vi "set operation mode.vi"(8 "error in (no error)":errorcluster, 11 "CCDCamera in":refnum<class "iKon-L.lvclass">) -> (0 "error out":errorcluster, 3 "CCDCamera out":refnum<class "iKon-L.lvclass">)   [LabVIEW 2018, in "iKon-L.lvclass"]
doc: "Set the camera configuration\n\nThis function records the given operating parameters in the camera. However, the parameters will only bewritten if their last value is different from the most recent one."
uses:
  iKon-L.lvclass
panel:
  out "x != y? 2":T1
  out "x != y?":T2
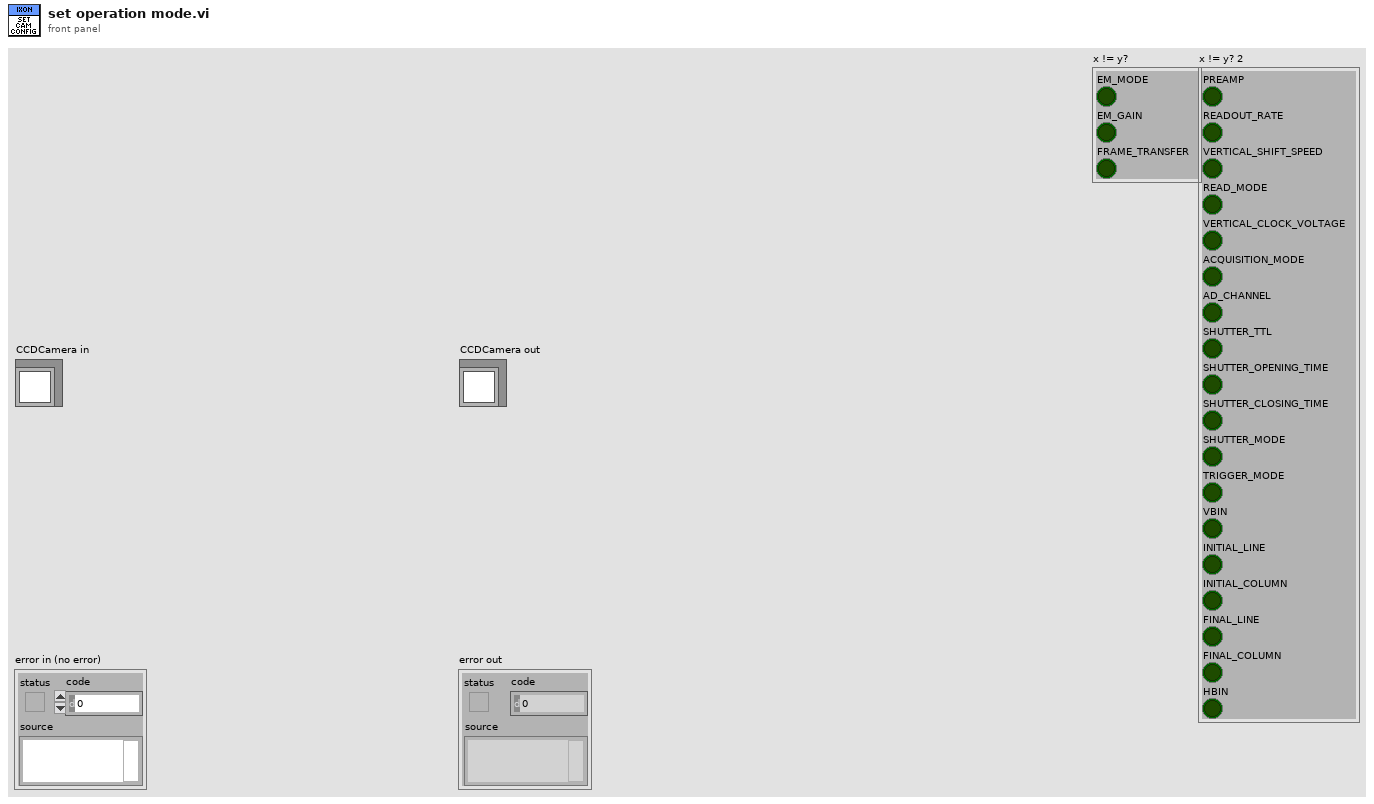
[diagram p1: front panel]
types:
  T1 = cluster{"PREAMP":bool, "READOUT_RATE":bool, "VERTICAL_SHIFT_SPEED":bool, "READ_MODE":bool, "VERTICAL_CLOCK_VOLTAGE":bool, "ACQUISITION_MODE":bool, "AD_CHANNEL":bool, "SHUTTER_TTL":bool, "SHUTTER_OPENING_TIME":bool, "SHUTTER_CLOSING_TIME":bool, "SHUTTER_MODE":bool, "TRIGGER_MODE":bool, "VBIN":bool, "INITIAL_LINE":bool, "INITIAL_COLUMN":bool, "FINAL_LINE":bool, "FINAL_COLUMN":bool, "HBIN":bool}
  T2 = cluster{"EM_MODE":bool, "EM_GAIN":bool, "FRAME_TRANSFER":bool}
  T3 = cluster{"PREAMP":u16, "READOUT_RATE":u16, "VERTICAL_SHIFT_SPEED":u16, "READ_MODE":u16, "VERTICAL_CLOCK_VOLTAGE":u16, "ACQUISITION_MODE":u16, "AD_CHANNEL":u16, "SHUTTER_TTL":u16, "SHUTTER_OPENING_TIME":u16, "SHUTTER_CLOSING_TIME":u16, "SHUTTER_MODE":u16, "TRIGGER_MODE":u16, "VBIN":u16, "INITIAL_LINE":u16, "INITIAL_COLUMN":u16, "FINAL_LINE":u16, "FINAL_COLUMN":u16, "HBIN":u16}
  T4 = cluster{"EM_MODE":u16, "EM_GAIN":u16, "FRAME_TRANSFER":bool}
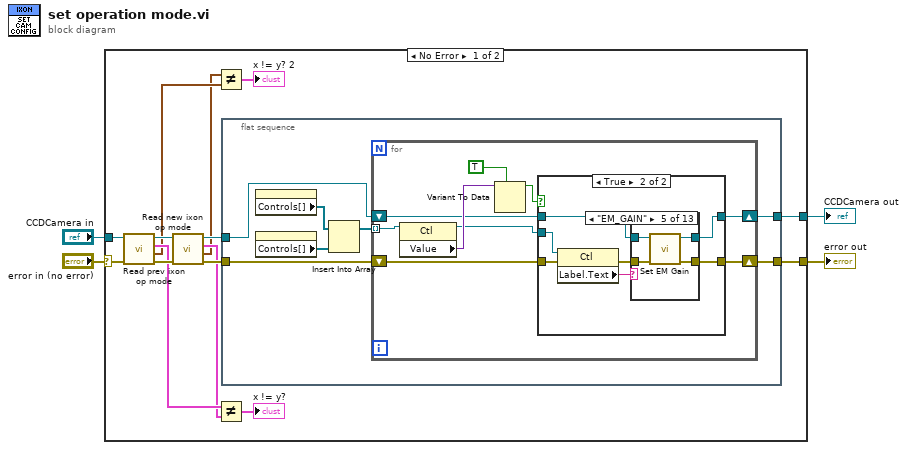
[diagram p0: block diagram]
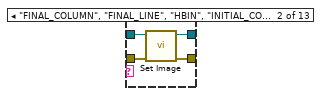
[diagram p4: hidden frame]
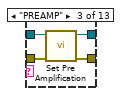
[diagram p5: hidden frame]
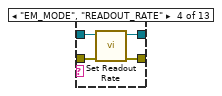
[diagram p6: hidden frame]
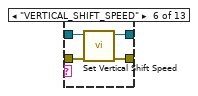
[diagram p7: hidden frame]
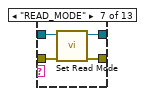
[diagram p8: hidden frame]
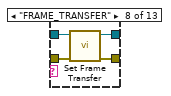
[diagram p9: hidden frame]
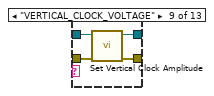
[diagram p10: hidden frame]
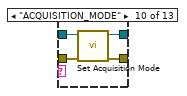
[diagram p11: hidden frame]
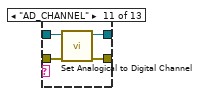
[diagram p12: hidden frame]
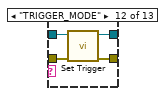
[diagram p13: hidden frame]
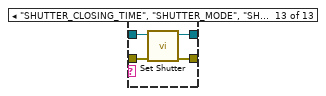
[diagram p14: hidden frame]
diagram:
  n1 = case shown="No Error" "error in (no error)" {
    selector: "error in (no error)" -> [w16 w95]
    tunnel: [w18 w95] -> w4
    tunnel: [w17 w94] -> w3
    tunnel: "CCDCamera in" -> [w15 w94]
    frame No Error {
      n2 = call-dynamic "Read prev ixon op mode.vi"("error in (no error)"=w16, "Sim_Ixon_Ultra in"=w15) -> ("error out"=w13:errorcluster, "prev operation mode"=w7:T3, "prev ixon op mode"=w10:T4, "Sim_Ixon_Ultra out"=w14:refnum<class "iKon-L.lvclass">)  [unwired: 6 in]
      n3 = call-dynamic "Read new ixon op mode.vi"("error in (no error)"=w13, "Sim_Ixon_Ultra in"=w14) -> ("error out"=w12:errorcluster, "new operation mode"=w6:T3, "new ixon op mode"=w9:T4, "Sim_Ixon_Ultra out"=w11:refnum<class "iKon-L.lvclass">)  [unwired: 6 in]
      n4 = Not Equal?(x=w6, y=w7) -> (x != y?=→"x != y? 2":T1)
      n5 = Not Equal?(x=w10, y=w9) -> (x != y?=→"x != y?":T2)
      n6 = flat-sequence {
        tunnel: w12 -> [w22]
        tunnel: [w25] -> w18
        tunnel: w11 -> [w24]
        tunnel: [w23] -> w17
        frame #0 {
          n7 = property on="x != y?" class="Clust (strict)"() -> ("Controls[]"=w20:refnum<vi>[])  [unwired: 2 in, 2 out]
          n8 = property on="x != y? 2" class="Clust (strict)"() -> ("Controls[]"=w19:refnum<vi>[])  [unwired: 2 in, 2 out]
          n9 = Insert Into Array(array=w20, new element=w19) -> (w21:refnum<vi>[])  [unwired: 1 in]
          n10 = for {
            shift-right: [w28] -> w25
            shift-left: w22 -> [w34]
            shift-right: [w29] -> w23
            shift-left: w24 -> [w30]
            tunnel: w21 -> [w27] mode=indexing
            n11 = property class="Ctl"(reference=w27) -> (reference out=w26:refnum<vi>, "Value"=w33:variant)  [unwired: 1 in, 1 out]
            n12 = Variant To Data(type=TRUE, Variant=w33) -> (data=w31:bool)  [unwired: 1 in, 1 out]
            n13 = case shown="True" w31 {
              tunnel: [w36 w38] -> w28
              tunnel: w34 -> [w36 w42]
              tunnel: w30 -> [w35 w41]
              tunnel: [w35 w40] -> w29
              tunnel: w26 -> [_ w37]
              frame False {
              }
              frame True {
                n14 = property class="Ctl"(reference=w37, error in=w42) -> (error out=w39:errorcluster, "Label.Text"=w43:string)  [unwired: 1 out]
                n15 = case shown="\"EM_GAIN\"" w43 {
                  tunnel: w41 -> [w45 w49 w53 w56 w61 w65 w69 w73 w76 w81 w85 w88 w93]
                  tunnel: [w45 w48 w52 w57 w60 w64 w68 w72 w77 w80 w84 w89 w92] -> w40
                  tunnel: w39 -> [w44 w47 w51 w55 w59 w63 w67 w71 w75 w79 w83 w87 w91]
                  tunnel: [w44 w46 w50 w54 w58 w62 w66 w70 w74 w78 w82 w86 w90] -> w38
                  frame "False", Default {
                  }
                  frame "FINAL_COLUMN", "FINAL_LINE", "HBIN", "INITIAL_COLUMN", "INITIAL_LINE", "VBIN" {
                    n16 = call-dynamic "Set Image.vi"("error in (no error)"=w47, "CCDCamera in"=w49) -> ("error out"=w46:errorcluster, "CCDCamera out"=w48:refnum<class "iKon-L.lvclass">)  [unwired: 8 in]
                  }
                  frame "PREAMP" {
                    n17 = call-dynamic "Set Pre Amplification.vi"("error in (no error)"=w51, "CCDCamera in"=w53) -> ("error out"=w50:errorcluster, "CCDCamera out"=w52:refnum<class "iKon-L.lvclass">)  [unwired: 8 in]
                  }
                  frame "EM_MODE", "READOUT_RATE" {
                    n18 = call-dynamic "Set Readout Rate.vi"("error in (no error)"=w55, "CCDCamera in"=w56) -> ("error out"=w54:errorcluster, "CCDCamera out"=w57:refnum<class "iKon-L.lvclass">)  [unwired: 8 in]
                  }
                  frame "EM_GAIN" {
                    n19 = call-dynamic "Set EM Gain.vi"("error in (no error)"=w59, "CCDCamera in"=w61) -> ("error out"=w58:errorcluster, "CCDCamera out"=w60:refnum<class "iKon-L.lvclass">)  [unwired: 8 in]
                  }
                  frame "VERTICAL_SHIFT_SPEED" {
                    n20 = call-dynamic "Set Vertical Shift Speed.vi"("error in (no error)"=w63, "CCDCamera in"=w65) -> ("error out"=w62:errorcluster, "CCDCamera out"=w64:refnum<class "iKon-L.lvclass">)  [unwired: 8 in]
                  }
                  frame "READ_MODE" {
                    n21 = call-dynamic "Set Read Mode.vi"("error in (no error)"=w67, "CCDCamera in"=w69) -> ("error out"=w66:errorcluster, "CCDCamera out"=w68:refnum<class "iKon-L.lvclass">)  [unwired: 8 in]
                  }
                  frame "FRAME_TRANSFER" {
                    n22 = call-dynamic "Set Frame Transfer.vi"("error in (no error)"=w71, "CCDCamera in"=w73) -> ("error out"=w70:errorcluster, "CCDCamera out"=w72:refnum<class "iKon-L.lvclass">)  [unwired: 8 in]
                  }
                  frame "VERTICAL_CLOCK_VOLTAGE" {
                    n23 = call-dynamic "Set Vertical Clock Amplitude.vi"("error in (no error)"=w75, "CCDCamera in"=w76) -> ("error out"=w74:errorcluster, "CCDCamera out"=w77:refnum<class "iKon-L.lvclass">)  [unwired: 8 in]
                  }
                  frame "ACQUISITION_MODE" {
                    n24 = call-dynamic "Set Acquisition Mode.vi"("error in (no error)"=w79, "CCDCamera in"=w81) -> ("error out"=w78:errorcluster, "CCDCamera out"=w80:refnum<class "iKon-L.lvclass">)  [unwired: 8 in]
                  }
                  frame "AD_CHANNEL" {
                    n25 = call-dynamic "Set Analogical to Digital Channel.vi"("error in (no error)"=w83, "CCDCamera in"=w85) -> ("error out"=w82:errorcluster, "CCDCamera out"=w84:refnum<class "iKon-L.lvclass">)  [unwired: 8 in]
                  }
                  frame "TRIGGER_MODE" {
                    n26 = call-dynamic "Set Trigger.vi"("error in (no error)"=w87, "CCDCamera in"=w88) -> ("error out"=w86:errorcluster, "CCDCamera out"=w89:refnum<class "iKon-L.lvclass">)  [unwired: 8 in]
                  }
                  frame "SHUTTER_CLOSING_TIME", "SHUTTER_MODE", "SHUTTER_OPENING_TIME", "SHUTTER_TTL" {
                    n27 = call-dynamic "Set Shutter.vi"("error in (no error)"=w91, "CCDCamera in"=w93) -> ("error out"=w90:errorcluster, "CCDCamera out"=w92:refnum<class "iKon-L.lvclass">)  [unwired: 8 in]
                  }
                }
              }
            }
          }
        }
      }
    }
    frame Error {
    }
  }
  "error out" <- w4
  "CCDCamera out" <- w3
